vi "Named Loggers.vi"() -> ()   [LabVIEW 2020]
uses:
  Source/LV Logging.lvlib
  Source/Type Defs/Debug Level.ctl
panel:
  in  "Log Path":path
  in  "error in (no error)":errorcluster
  in  "Debug Level":T1
  out "error out":errorcluster
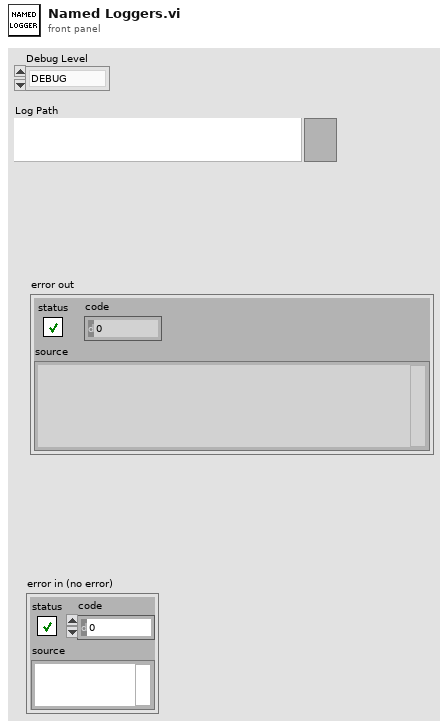
[diagram p1: front panel]
types:
  T1 = typedef "LV Logging.lvlib/Debug Level.ctl" = enum16{"DEBUG", "INFO", "WARN", "ERROR", "FATAL"}
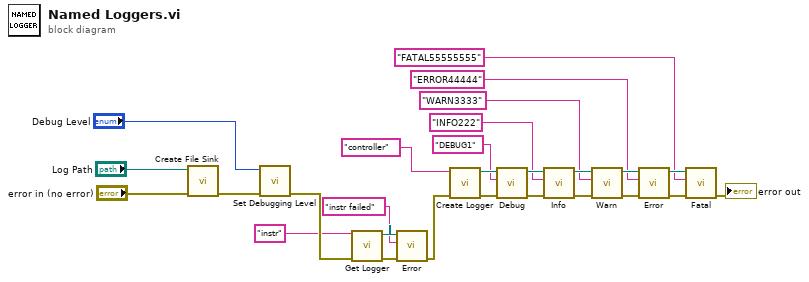
[diagram p0: block diagram]
diagram:
  n1 = call "Create File Sink.vi"("error in (no error)"="error in (no error)", "Path"="Log Path") -> ("error out"=w26:errorcluster)  [unwired: 9 in]
  n2 = call "Set Debugging Level.vi"("error in (no error)"=w26, "Debug Level in"="Debug Level") -> ("error out"=w24:errorcluster)  [unwired: 9 in]
  n3 = call "Get Logger.vi"("error in (no error)"=w24, "Name"="instr") -> ("error out"=w6:errorcluster, "Logger out"=w5:refnum<class "Logger.lvclass">)  [unwired: 8 in]
  n4 = call "Error.vi"("error in (no error)"=w6, "Log Text"="instr failed", "Logger in"=w5) -> ("error out"=w4:errorcluster)  [unwired: 7 in, 1 out]
  n5 = call "Create Logger.vi"("error in (no error)"=w4, "Name"="controller") -> ("error out"=w22:errorcluster, "Logger out"=w21:refnum<class "Logger.lvclass">)  [unwired: 8 in]
  n6 = call "Debug.vi"("error in (no error)"=w22, "Log Text"="DEBUG1", "Logger in"=w21) -> ("error out"=w19:errorcluster, "Logger out"=w20:refnum<class "Logger.lvclass">)  [unwired: 7 in]
  n7 = call "Info.vi"("error in (no error)"=w19, "Log Text"="INFO222", "Logger in"=w20) -> ("error out"=w18:errorcluster, "Logger out"=w17:refnum<class "Logger.lvclass">)  [unwired: 7 in]
  n8 = call "Warn.vi"("error in (no error)"=w18, "Log Text"="WARN3333", "Logger in"=w17) -> ("error out"=w15:errorcluster, "Logger out"=w16:refnum<class "Logger.lvclass">)  [unwired: 7 in]
  n9 = call "Error.vi"("error in (no error)"=w15, "Log Text"="ERROR44444", "Logger in"=w16) -> ("error out"=w14:errorcluster, "Logger out"=w13:refnum<class "Logger.lvclass">)  [unwired: 7 in]
  n10 = call "Fatal.vi"("error in (no error)"=w14, "Log Text"="FATAL55555555", "Logger in"=w13) -> ("error out"=→"error out":errorcluster)  [unwired: 7 in, 1 out]
